vi "SET_MODE.vi"(9 "Flight Mode":T1, 10 "base_mode":T2(ring), 11 "target_system":u8=1) -> (3 "MAVLink Message":u8[](array[numeric]))   [LabVIEW 2014]
uses:
  Controls/MAVLink Flight modes.ctl
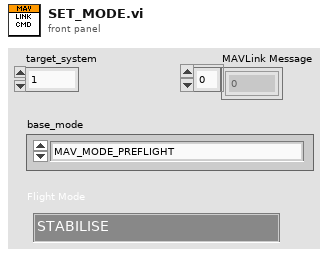
[diagram p1: front panel]
types:
  T1 = typedef "MAVLink Flight modes.ctl" = enum32{"STABILISE", "ACRO", "ALT HOLD", "AUTO", "GUIDED", "LOITER", "RTL", "CIRCLE", "UNKNOWN1", "LAND", "OF LOITER", "DRIFT", "UNKNOWN2", "SPORT", "FLIP", "AUTO TUNE", "POS HOLD", "BRAKE"}
  T2 = enum16{"MAV_MODE_PREFLIGHT", "MAV_MODE_STABILIZE_DISARMED", "MAV_MODE_STABILIZE_ARMED", "MAV_MODE_MANUAL_DISARMED", "MAV_MODE_MANUAL_ARMED", "MAV_MODE_GUIDED_DISARMED", "MAV_MODE_GUIDED_ARMED", "MAV_MODE_AUTO_DISARMED", "MAV_MODE_AUTO_ARMED", "MAV_MODE_TEST_DISARMED", "MAV_MODE_TEST_ARMED"}
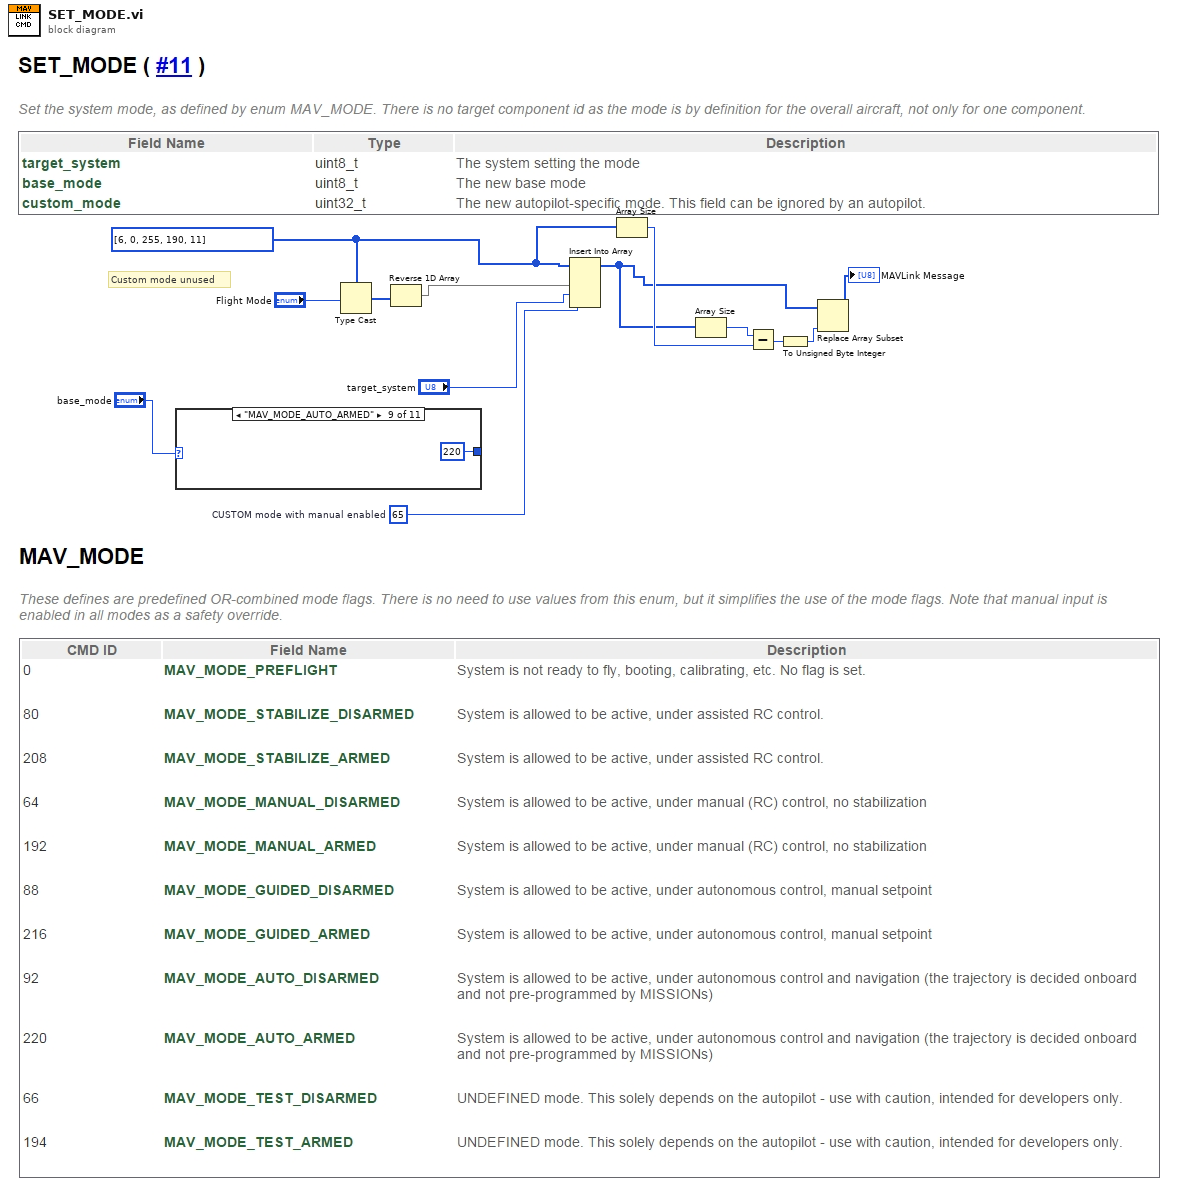
[diagram p0: block diagram]
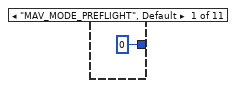
[diagram p2: hidden frame]
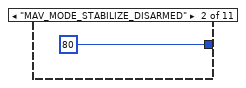
[diagram p3: hidden frame]
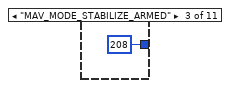
[diagram p4: hidden frame]
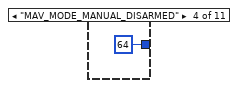
[diagram p5: hidden frame]
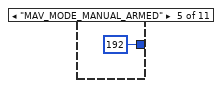
[diagram p6: hidden frame]
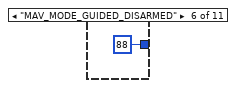
[diagram p7: hidden frame]
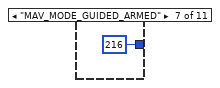
[diagram p8: hidden frame]
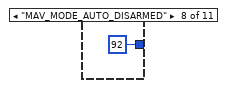
[diagram p9: hidden frame]
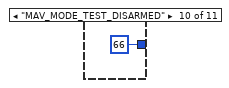
[diagram p10: hidden frame]
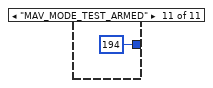
[diagram p11: hidden frame]
diagram:
  w1 = u8 65  # CUSTOM mode with manual enabled
  w4 = u8[] [6, 0, 255, 190, 11]
  # "Custom mode unused"
  n1 = case shown="\"MAV_MODE_AUTO_ARMED\"" "base_mode" {
    tunnel: [u8 0 ("new element/subarray") u8 80 ("new element/subarray") u8 208 ("new element/subarray") u8 64 ("new element/subarray") u8 192 ("new element/subarray") u8 88 ("new element/subarray") u8 216 ("new element/subarray") u8 92 ("new element/subarray") u8 220 ("new element/subarray") u8 66 ("new element/subarray") u8 194 ("new element/subarray")] -> _
    frame "MAV_MODE_PREFLIGHT", Default {
    }
    frame "MAV_MODE_STABILIZE_DISARMED" {
    }
    frame "MAV_MODE_STABILIZE_ARMED" {
    }
    frame "MAV_MODE_MANUAL_DISARMED" {
    }
    frame "MAV_MODE_MANUAL_ARMED" {
    }
    frame "MAV_MODE_GUIDED_DISARMED" {
    }
    frame "MAV_MODE_GUIDED_ARMED" {
    }
    frame "MAV_MODE_AUTO_DISARMED" {
    }
    frame "MAV_MODE_AUTO_ARMED" {
    }
    frame "MAV_MODE_TEST_DISARMED" {
    }
    frame "MAV_MODE_TEST_ARMED" {
    }
  }
  n2 = Type Cast(type=w4, x="Flight Mode") -> (*(type *) &x=w3:u8[])
  n3 = Reverse 1D Array(array=w3) -> (reversed array=w2:u8[])
  n4 = Insert Into Array(array=w4, new element #1=w2, new element #2="target_system", new element #3=w1) -> (w10:u8[])  [unwired: 1 in]
  n5 = Array Size(array=w4) -> (size(s)=w11:i32)
  n6 = Array Size(array=w10) -> (size(s)=w12:i32)
  n7 = Subtract(x=w12, y=w11) -> (x-y=w8:i32)
  n8 = To Unsigned Byte Integer(number=w8) -> (unsigned 8bit integer=w7:u8)
  n9 = Replace Array Subset(array=w10, new element=w7) -> (→"MAVLink Message":u8[])  [unwired: 1 in]
